vi "SAOMM-SendGET.vi"(0 "PRAMMS-COMM IN":refnum<visa-resource-name>="COM4", 1 "Bool Refnum":refnum<vi>, 2 "MessageType":cluster{string[], u32[]}={["emtError", "emtAreYouThere", "emtAcknowledgment", "emtGetClientType", "emtClientType", "emtGetImageExposureTime", "emtGetOptimalExposureTime", "emtGetImageEMGain", "emtGetFPGACtrl", "emtGetImageWidth", "emtGetImageHeight", "emtGetImageBinning", "emtGetImageDisplayFrameRate", "emtGetROIWidth", "emtGetROIHeight", "emtGetROIXOffset", "emtGetROIYOffset", "emtGetTelescopeServoLevel", "emtGetIsAcquisitionStarted", "emtGetFalconImage", "emtGetProcessedFalconImage", "emtSetImageExposureTime", "emtSetOptimalExposureTime", "emtSetImageEMGain", "emtSetFPGACtrl", "emtSetImageWidth", "emtSetImageHeight", "emtSetImageBinning", "emtSetImageDisplayFrameRate", "emtSetROIWidth", "emtSetROIHeight", "emtSetROIXOffset", "emtSetROIYOffset", "emtSetTelescopeServoLevel", "emtStartAcquisition", "emtStopAcquisition", "emtAcquisitionStarted", "emtAcquisitionStopped", "emtImageExposureTime", "emtOptimalExposureTime", "emtImageEMGain", "emtFPGACtrl", "emtImageWidth", "emtImageHeight", "emtImageBinning", "emtImageDisplayFrameRate", "emtROIWidth", "emtROIHeight", "emtROIXOffset", "emtROIYOffset", "emtTelescopeServoLevel", "emtIsAcquisitionStarted", "emtFalconImage", "emtProcessedFalconImage", "emtGetXAxis", "emtGetYAxis", "emtGetZAxis", "emtGetUAxis", "emtGetVAxis", "emtGetWAxis", "emtGetVelocity", "emtGetMoveIncrement", "emtGetXAxisOffset", "emtGetYAxisOffset", "emtGetZAxisOffset", "emtGetUAxisOffset", "emtGetVAxisOffset", "emtGetWAxisOffset", "emtSetXAxis", "emtSetYAxis", "emtSetZAxis", "emtSetUAxis", "emtSetVAxis", "emtSetWAxis", "emtSetVelocity", "emtSetMoveIncrement", "emtSetXAxisOffset", "emtSetYAxisOffset", "emtSetZAxisOffset", "emtSetUAxisOffset", "emtSetVAxisOffset", "emtSetWAxisOffset", "emtMoveTo", "emtHalt", "emtApplyAxesOffsets", "emtMoveStarted", "emtMoveStopped", "emtMoving"], [1, 2, 3, 4, 5, 1001, 1002, 1003, 1004, 1005, 1006, 1007, 1008, 1009, 1010, 1011, 1012, 1013, 1014, 1070, 1071, 1101, 1102, 1103, 1104, 1105, 1106, 1107, 1108, 1109, 1110, 1111, 1112, 1113, 1130, 1131, 1150, 1151, 1201, 1202, 1203, 1204, 1205, 1206, 1207, 1208, 1209, 1210, 1211, 1212, 1213, 1214, 1270, 1271, 2001, 2002, 2003, 2004, 2005, 2006, 2007, 2008, 2009, 2010, 2011, 2012, 2013, 2014, 2101, 2102, 2103, 2104, 2105, 2106, 2107, 2108, 2109, 2110, 2111, 2112, 2113, 2114, 2130, 2131, 2138, 2150, 2151, 2152]}, 7 "Signature":u32=1886544237, 11 "Error IN":errorcluster, 13 "Active GET":string) -> (4 "PRAMMS-COMM OUT":refnum<visa-resource-name>="COM4", 15 "Error OUT":errorcluster)   [LabVIEW 2019]
panel:
  out "bytes written":i32
  out "TypeEnum":u32[](array[numeric])=[1, 2, 3, 4, 5, 1001, 1101, 1201, 1002, 1102, 1202, 1003, 1103, 1203, 1004, 1104, 1204, 1005, 1105, 1205, 1006, 1106, 1206, 1007, 1107, 1207, 1008, 1108, 1208, 1009, 1109, 1209, 1010, 1110, 1210, 1011, 1111, 1211, 1012, 1112, 1212, 1130, 1131, 1150, 1151, 1070, 1270]
  out "CommandEnum":string[](array[string])=["emtError", "emtAreYouThere", "emtAcknowledgment", "emtGetClientType", "emtClientType", "emtGetImageExposureTime", "emtSetImageExposureTime", "emtImageExposureTime", "emtGetOptimalExposureTime", "emtSetOptimalExposureTime", "emtOptimalExposureTime", "emtGetImageEMGain", "emtSetImageEMGain", "emtImageEMGain", "emtGetFPGACtrl", "emtSetFPGACtrl", "emtFPGACtrl", "emtGetImageWidth", "emtSetImageWidth", "emtImageWidth", "emtGetImageHeight", "emtSetImageHeight", "emtImageHeight", "emtGetImageBinning", "emtSetImageBinning", "emtImageBinning", "emtGetImageDisplayFrameRate", "emtSetImageDisplayFrameRate", "emtImageDisplayFrameRate", "emtGetROIWidth", "emtSetROIWidth", "emtROIWidth", "emtGetROIHeight", "emtSetROIHeight", "emtROIHeight", "emtGetROIXOffset", "emtSetROIXOffset", "emtROIXOffset", "emtGetROIYOffset", "emtSetROIYOffset", "emtROIYOffset", "emtStartAcquisition", "mtStopAcquisition", "emtAcquisitionStarted", "emtAcquisitionStopped", "emtGetFalconImage", "emtFalconImage"]
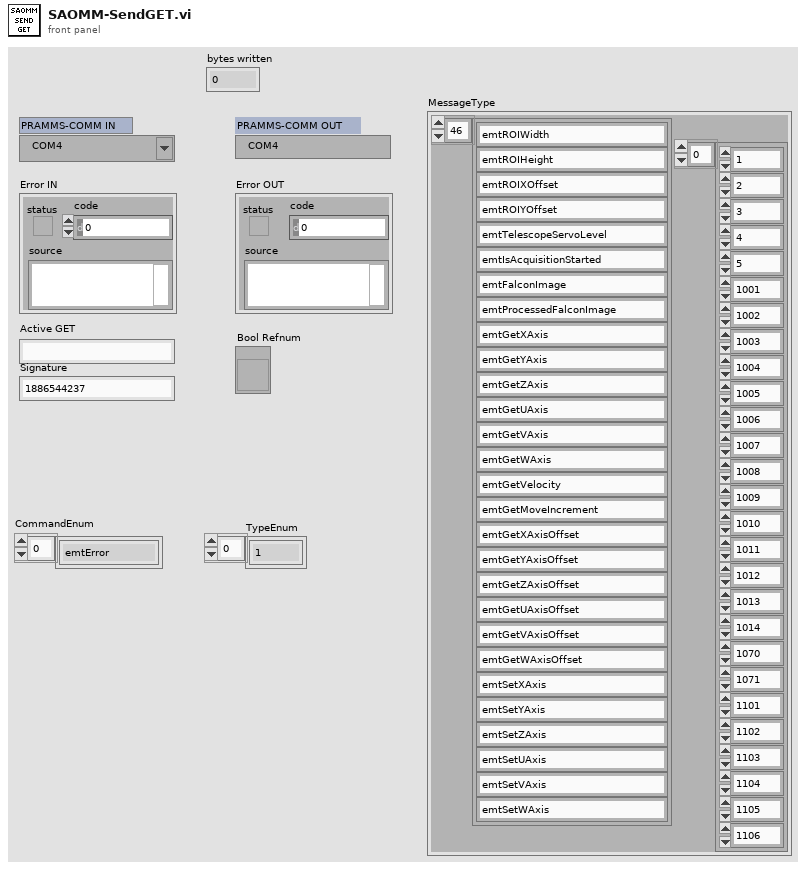
[diagram p1: front panel]
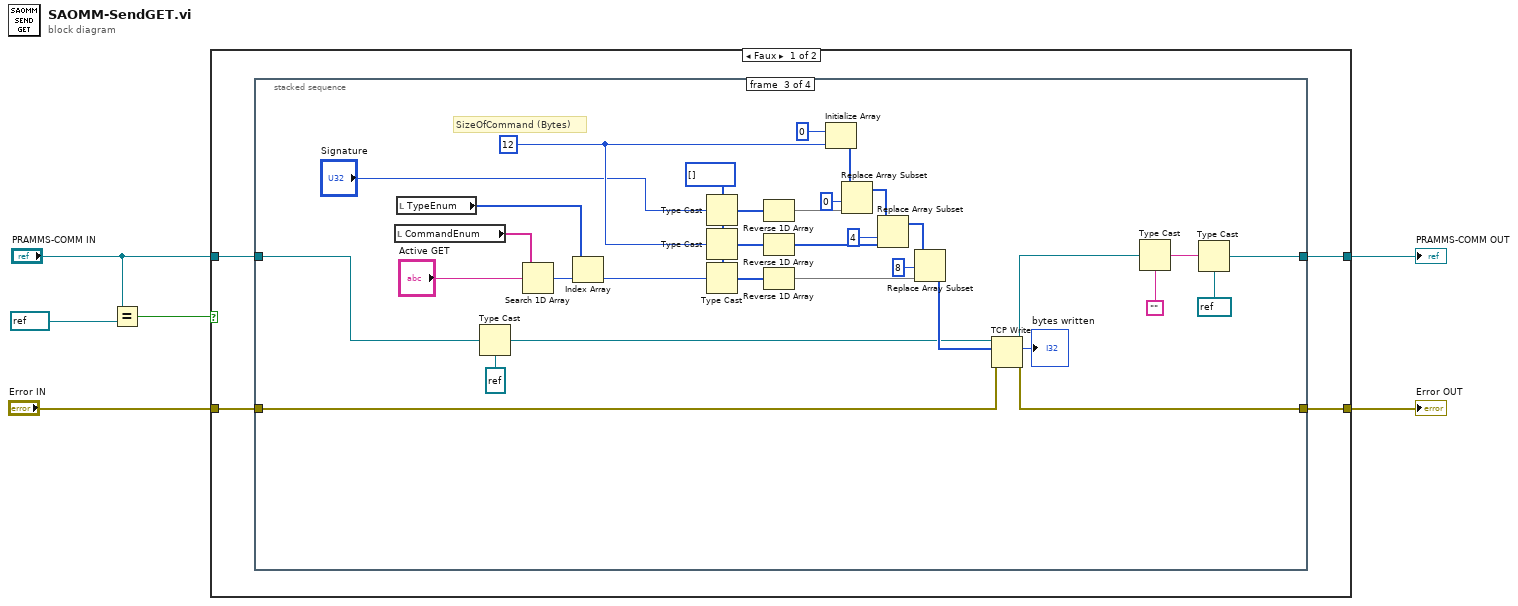
[diagram p0: block diagram]
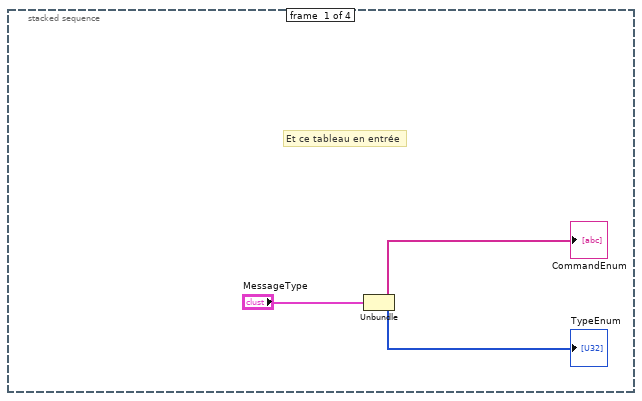
[diagram p2: hidden frame]
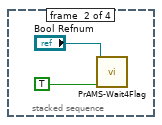
[diagram p3: hidden frame]
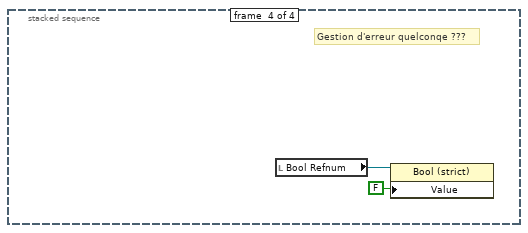
[diagram p4: hidden frame]
diagram:
  n1 = Equal?(x="PRAMMS-COMM IN", y=refnum<visa-resource-name> "-1") -> (x = y?=w5:bool)
  n2 = case shown="Faux" w5 {
    tunnel: "PRAMMS-COMM IN" -> [w9 w51]
    tunnel: "Error IN" -> [w10 w52]
    tunnel: [w7 w52] -> w2
    tunnel: [w8 w51] -> w1
    frame False {
      n3 = stacked-sequence {
        tunnel: w10 -> [_ _ w26 _]
        tunnel: w9 -> [_ _ w25 _]
        tunnel: [_ _ w22 _] -> w8
        tunnel: [_ _ w18 _] -> w7
        frame #0 {
          # "Et ce tableau en entrée"
          n4 = Unbundle("MessageType") -> (→"CommandEnum":string[], →"TypeEnum":u32[])
        }
        frame #1 {
          n5 = call "PrAMS-Wait4Flag.vi"("Raise Flag ?"=TRUE, "Ctl Refnum IN"="Bool Refnum") -> ()  [unwired: 8 in, 2 out]
        }
        frame #2 {
          w30 = 12 ("dimension size")
          w44 = u8[] []
          # "SizeOfCommand (Bytes)"
          n6 = local read "CommandEnum"() -> (w47:string[])
          n7 = local read "TypeEnum"() -> (w45:u32[])
          n8 = Type Cast(type=refnum<k5> refnum ("connection ID out"), x=w25) -> (*(type *) &x=w27:refnum<k5>)
          n9 = Search 1D Array(1D array=w47, element="Active GET") -> (index of element=w46:i32)  [unwired: 1 in]
          n10 = Index Array(array=w45, index=w46) -> (element=w29:u32)
          n11 = Type Cast(type=w44, x="Signature") -> (*(type *) &x=w31:u8[])
          n12 = Type Cast(type=w44, x=w30) -> (*(type *) &x=w43:u8[])
          n13 = Type Cast(type=w44, x=w29) -> (*(type *) &x=w42:u8[])
          n14 = Reverse 1D Array(array=w31) -> (reversed array=w37:u8[])
          n15 = Reverse 1D Array(array=w43) -> (reversed array=w33:u8[])
          n16 = Reverse 1D Array(array=w42) -> (reversed array=w32:u8[])
          n17 = Initialize Array(u8 0, w30) -> (w40:u8[])
          n18 = Replace Array Subset(array=w40, new element=w37, index=0) -> (w39:u8[])
          n19 = Replace Array Subset(array=w39, new element=w33, index=4) -> (w38:u8[])
          n20 = Replace Array Subset(array=w38, new element=w32, index=8) -> (w28:u8[])
          n21 = TCP Write(connection ID=w27, data in=w28, error in (no error)=w26) -> (connection ID out=w19:refnum<k5>, bytes written=→"bytes written":i32, error out=w18:errorcluster)  [unwired: 1 in]
          n22 = Type Cast(type="", x=w19) -> (*(type *) &x=w23:string)
          n23 = Type Cast(type=refnum<visa-resource-name> refnum ("y"), x=w23) -> (*(type *) &x=w22:refnum<visa-resource-name>)
        }
        frame #3 {
          # "Gestion d'erreur quelconqe ???"
          n24 = local read "Bool Refnum"() -> (w50:refnum<vi>)
          n25 = property class="Bool (strict)"(reference=w50, "Value"=FALSE) -> ()  [unwired: 1 in, 2 out]
        }
      }
    }
    frame True {
    }
  }
  "PRAMMS-COMM OUT" <- w1
  "Error OUT" <- w2
